vi "Swerve Drive Controller.vi"(8 "error in":errorcluster) -> ()   [LabVIEW 2016]
doc: "This VI executes continuously carrying out the current operation and responding to updates or new operations. It will often contain the timing or control code that is difficult to place directly in TeleOp. This VI generally opens all sensors and motors and isolates the rest of the robot code from knowing how the operations are carried out."
uses:
  Swerve Drive Setpoints.ctl
  Swerve Drive Operations.ctl
  <vilib>/Rock Robotics/WPI/ThirdParty/CanMotor/TalonSRX/WPI_CANTalonSRX_APIControlMode.ctl
  <vilib>/Rock Robotics/Network Tables/NT Read Boolean.vi
  Framework/Robot Global Data.vi
  Support Code/Team900-VIs/Team900SwerveDrive/SwerveDriveFuse.vi
  Swerve Drive Published Globals.vi
  <vilib>/Rock Robotics/Network Tables/SD Read Boolean.vi
  <vilib>/Rock Robotics/Network Tables/NT Read Numeric Array.vi
  Support Code/Team900-VIs/Team900SwerveDrive/SwerveGlobalData.vi
  Support Code/Team900-VIs/Team900SwerveDrive/Team900SwerveDrive.lvlib
  Support Code/Team900-VIs/navX Library v2/navX Library v2.lvlib
panel:
  in  "Reset Offsets":bool
  out "Loop Time":u32
  in  "Max Wheel Speed":dbl=20000.0
  in  "Distance PID gains":T1={"proportional gain (Kc)"=0.0125, "integral time (Ti, min)"=0.0, "derivative time (Td, min)"=0.00225} {"derivative time (Td, min)" format="%_5g"; "integral time (Ti, min)" format="%_5g"; "proportional gain (Kc)" format="%_5g"}
  in  "Face PID Gains":T1={"proportional gain (Kc)"=0.275, "integral time (Ti, min)"=0.0, "derivative time (Td, min)"=0.006} {"derivative time (Td, min)" format="%.3f"; "integral time (Ti, min)" format="%.3f"; "proportional gain (Kc)" format="%.3f"}
  out "Speed Chart":cluster{dbl, "Encoder Velocity":dbl}[](graph)
  out "Current\nCmd":string
  # "Tip: It may be helpful to observe inputs and sensor values.\nYou may also want to display tuning or debugging controls."
  # "To reset offsets, deploy the code, point the wheels facing toward the right of the robot, and the big gear facing to the back of the robot."
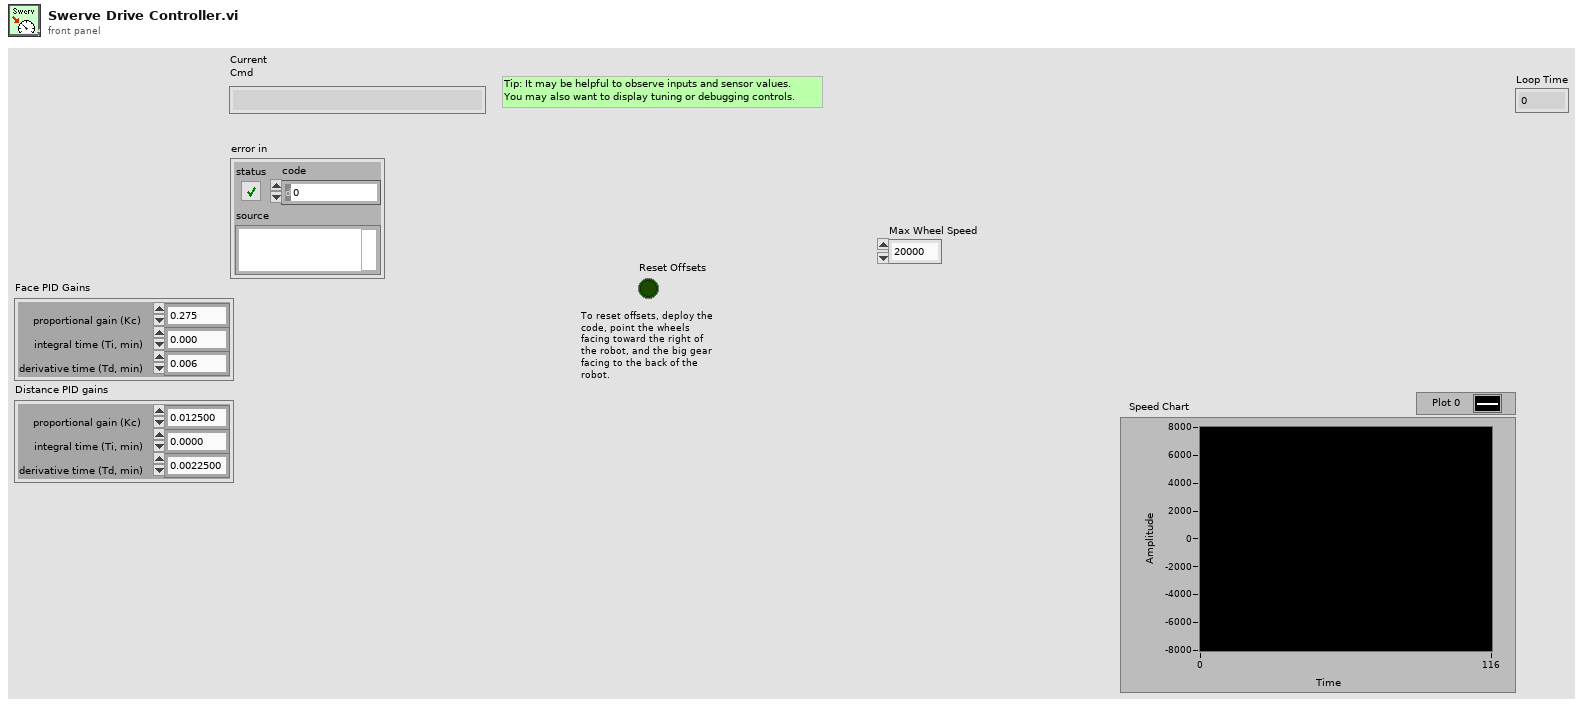
[diagram p1: front panel]
types:
  T1 = cluster{"proportional gain (Kc)":dbl, "integral time (Ti, min)":dbl, "derivative time (Td, min)":dbl}
  T2 = typedef "Swerve Drive Setpoints.ctl" = cluster{"Operation":T3, "Duration":dbl, "Strafe Joystick Axes":cluster{"X":dbl, "Y":dbl}, "Face Joystick Axes":cluster{"X":dbl, "Y":dbl}, "Trigger Axes":cluster{"Left":dbl, "Right":dbl}, "Coordinates":cluster{"X":dbl, "Y":dbl, "Angle":dbl}, "Speed Mode?":bool}
  T3 = typedef "Swerve Drive Operations.ctl" = enum16{"Reserve", "Read Current", "Immediate", "Go to Coordinate", "Drive Immediate (Turn Speed/Face and Stafe)"}
  T4 = typedef "Command Status Info.ctl" = cluster{"Name":string, "Status":T5, "notifier out":T6}
  T5 = typedef "Completion Status.ctl" = enum16{"Successful", "Aborted", "Incomplete"}
  T6 = typedef "Completion Notifier.ctl" = refnum<notifier>
  T7 = cluster{"Default Command":T2, "Command Timing":cluster{"Start Time (ms)":u32, "Iterations":i32}, "Command Arguments":cluster{"Command Info":T4, "Description":string, "Default Command":T2, "notifier out":refnum<notifier>, "Subsystem Name":string}}
  T8 = typedef "WPI_MotorControlDeviceRef.ctl" = cluster{"DeviceStatus":errorcluster, "Type":T9, "PWM":cluster{"PWM Channel":T10, "DeadBand":T11}, "CAN":cluster{"Device Number":u8, "SetOutput VI Ref":variant, "GetOutput VI Ref":variant, "Enable VI Ref":variant, "Disable VI Ref":variant, "Data":variant}, "Invert":bool}
  T9 = typedef "WPI_MotorControlType.ctl" = enum16{"PWM", "CAN"}
  T10 = typedef "FPGA_DIOPWMChannel.ctl" = enum8{"PWM 0", "PWM 1", "PWM 2", "PWM 3", "PWM 4", "PWM 5", "PWM 6", "PWM 7", "PWM 8", "PWM 9", "PWM MXP 0", "PWM MXP 1", "PWM MXP 2", "PWM MXP 3", "PWM MXP 4", "PWM MXP 5", "PWM MXP 6", "PWM MXP 7", "PWM MXP 8", "PWM MXP 9", "Invalid"}
  T11 = typedef "WPI_PWMDeadband.ctl" = cluster{"Name":string, "maxPositivePwm":i32, "minPositivePwm":i32, "centerPwm":i32, "maxNegativePwm":i32, "minNegativePwm":i32, "angularRange":u16}
  T12 = typedef "navX Library v2.lvlib/Z900_navX_DeviceTypeDef.ctl" = cluster{"Interface":cluster{"Protocol":T13, "Update Rate (4Hz-60Hz)":u8, "navX Open TypeDef":variant}, "Notify Packet":refnum<notifier>, "Loop VI Refnum":refnum<vi>, "Ready to Close Occurrence Refnum":refnum<k4>}
  T13 = typedef "navX Library v2.lvlib/Z900_navX_ProtocolTypeDef.ctl" = enum16{"SERIAL", "I2C", "SPI"}
  T14 = cluster{"Yaw":dbl, "Roll":dbl, "Pitch":dbl, "Heading":dbl, "Fused Heading":dbl}
  T15 = typedef "WPI_CANTalonSRX_GlobalStatus.ctl" = cluster{"Applied Throttle":dbl, "Module Enabled":bool, "CAN Error":errorcluster, "Closed Loop Error":dbl, "Forward Limit Switch Closed":bool, "Reverse Limit Switch Closed":bool, "Sensor Position":dbl, "Sensor Velocity":dbl, "Current":dbl, "Sticky Fault - Over Temp":bool, "Sticky Fault - Under Voltage":bool, "Sticky Fault - Forward Limit":bool, "Sticky Fault - Reverse Limit":bool, "Sticky Fault - Forward Soft Limit":bool, "Sticky Fault - Reverse Soft Limit":bool, "Brake is Enabled":bool, "Encoder Position":dbl, "Encoder Velocity":dbl, "Encoder Index Count":dbl, "Encoder A Pin State":bool, "Encoder B Pin State":bool, "Encoder Index Pin State":bool, "Analog In":dbl, "Analog In Velocity":dbl, "Temperature (C)":dbl, "Battery Voltage":dbl, "Control 5 Is Supported":bool, "Current Profile Slot Select":dbl, "Pos Div 8":bool, "Vel Div 4":bool, "Pulse Width Position":i32, "Pulse Width Velocity":i32, "Pulse Width Rise To Rise (us)":i32, "Pulse Width Rise To Fall (us)":i32, "Mot Prof Active Is Under Run":bool, "Mot Prof Active Has Under Run":bool, "Mot Prof Active Is Last":bool, "Mot Prof Active Velocity Only":bool, "Mot Prof Active Is Valid":bool, "Mot Prof Buffer Is Full":bool, "Mot Prof Active Profile Slot Select":i32, "Mot Prof NextID":i32, "Mot Prof Count":i32, "Mot Prof Active Velocity":dbl, "Mot Prof Active Position":dbl, "Mot Prof Output Enable":i32}
  T16 = cluster{"[0]":dbl, "[1]":dbl, "[2]":dbl, "[3]":dbl}
  T17 = cluster{"Numeric Array[0]":dbl, "Numeric Array[1]":dbl, "Numeric Array[2]":dbl}
  T18 = typedef "WPI_CANTalonSRX_APIControlMode.ctl" = enum8{"Percent VBus", "Speed", "Position", "Slave", "Unchanged / Invalid", "Voltage Compensation", "Current", "Motion Profile"}
  T19 = cluster{"Steering Motor Refs[0]":T8, "Steering Motor Refs[1]":T8, "Steering Motor Refs[2]":T8, "Steering Motor Refs[3]":T8}
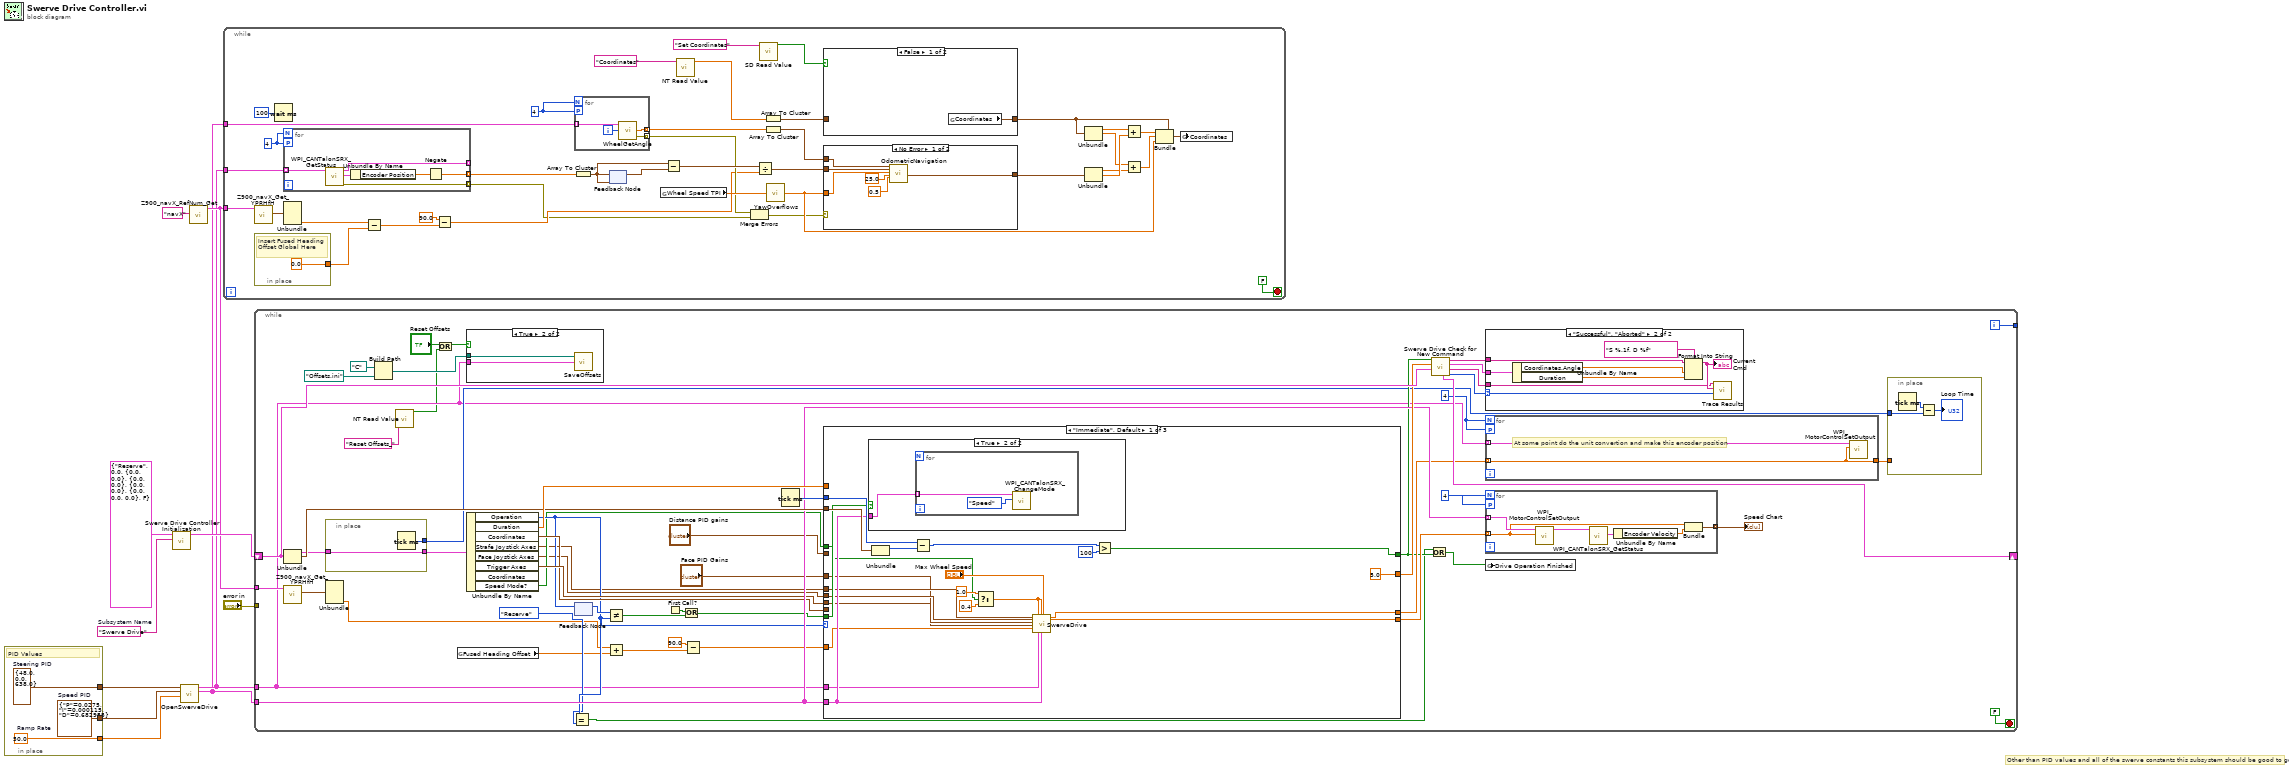
[diagram p0: block diagram]
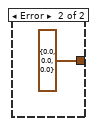
[diagram p2: hidden frame]
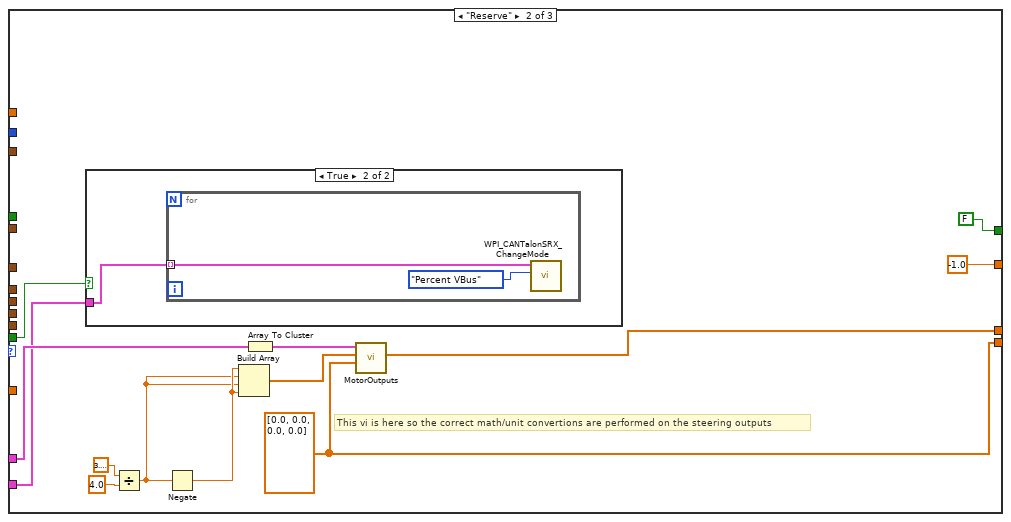
[diagram p7: hidden frame]
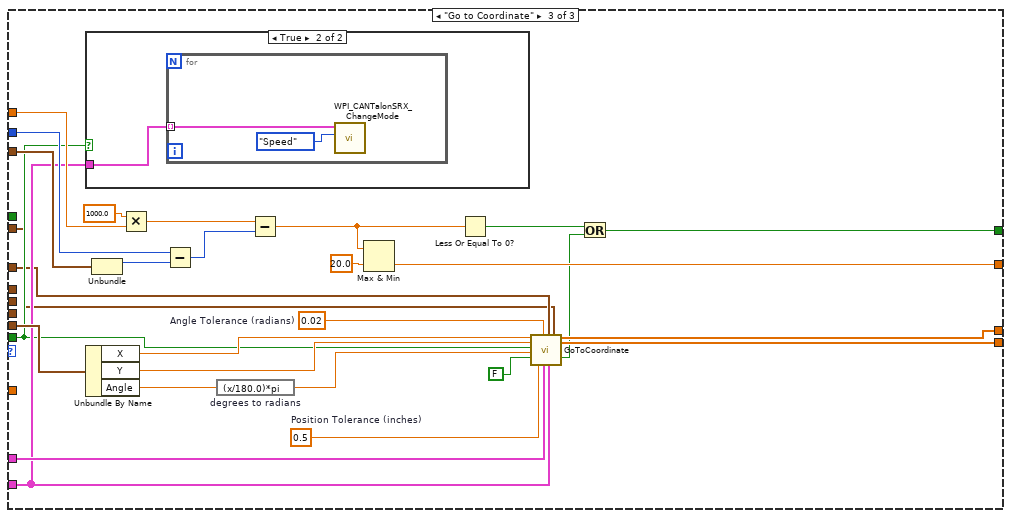
[diagram p9: hidden frame]
diagram:
  w1 = "Swerve Drive"  # Subsystem Name
  # "Other than PID values and all of the swerve constants this subsystem should be good to go"
  n1 = in-place {
    in-place-border: [w13] -> w9
    in-place-border: [w12] -> w8
    in-place-border: [w14] -> w4
    w14 = 50.0  # Ramp Rate
    w12 = cluster{"P":dbl, "I":dbl, "D":dbl} {"P"=0.0275, "I"=0.000115, "D"=0.682955}  # Speed PID
    w13 = cluster{"P":dbl, "I":dbl, "D":dbl} {"P"=48.0, "I"=0.0, "D"=638.0}  # Steering PID
    # "PID Values"
  }
  n2 = call "Swerve Drive Controller Initialization.vi"("Subsystem Name"=w1, "Default Command"=T2 {"Operation"=enum."Reserve", "Duration"=0.0, "Strafe Joystick Axes"={"X"=0.0, "Y"=0.0}, "Face Joystick Axes"={"X"=0.0, "Y"=0.0}, "Trigger Axes"={"Left"=0.0, "Right"=0.0}, "Coordinates"={"X"=0.0, "Y"=0.0, "Angle"=0.0}, "Speed Mode?"=FALSE}) -> ("Command Info"=w10:T7)  [unwired: 9 in]
  n3 = call "OpenSwerveDrive.vi"("Ramp Rate"=w4, "Speed PID"=w8, "Steering PID"=w9) -> ("Speed Motor Refs"=w2:T8[], "Steering Motor Refs"=w3:T8[])  [unwired: 4 in, 1 out]
  n4 = call "Z900_navX_RefNum_Get.vi"("refnum name"="navX") -> ("navX Device"=w6:T12)  [unwired: 9 in, 1 out]
  n5 = while {
    tunnel: w6 -> [w52]
    tunnel: w3 -> [w50]
    tunnel: w2 -> [w49]
    stop <- FALSE stop-if-true
    w23 = 4
    w24 = 4
    n6 = call "Z900_navX_Get_YPRHfH.vi"("navX Device"=w52) -> ("YRPHfH"=w48:T14)  [unwired: 7 in, 3 out]
    n7 = in-place {
      in-place-border: [0.0] -> w46
      # "Insert Fused Heading Offset Global Here"
    }
    n8 = Wait (ms)(milliseconds to wait=u32 100) -> ()  [unwired: 1 out]
    n9 = for {
      N: w24 -> [_]
      tunnel: [w68] -> _ mode=indexing
      tunnel: [w70] -> w34 mode=indexing
      workers-P: w24 -> [_]
      tunnel: w50 -> [w67] mode=indexing
      tunnel: [w66] -> w28 mode=indexing
      n10 = call <vilib>:"WPI_CANTalonSRX_GetStatus.vi"("CAN Talon SRX Ref"=w67) -> ("error out"=w70:errorcluster, "Talon SRX Status"=w69:T15, "CAN Talon SRX Ref"=w68:T8)  [unwired: 8 in]
      n11 = Unbundle By Name(w69) -> ("Encoder Position"=w65:dbl)
      n12 = Negate(x=w65) -> (-x=w66:dbl)
    }
    n13 = Unbundle(w48) -> ("Fused Heading"=w47:dbl)  [unwired: 4 out]
    n14 = Subtract(x=w47, y=w46) -> (x-y=w18:dbl)
    n15 = Subtract(x=90.0, y=w18) -> (x-y=w40:dbl)
    n16 = for {
      N: w23 -> [_]
      workers-P: w23 -> [_]
      tunnel: [w56] -> w27 mode=indexing
      tunnel: w49 -> [w55] mode=indexing
      tunnel: [w54] -> w25 mode=indexing
      i -> [w57]
      n17 = call "WheelGetAngle.vi"("Wheel"=w57, "CAN Talon SRX Ref"=w55) -> ("error out"=w56:errorcluster, "Sensor Position (rad)"=w54:dbl)  [unwired: 1 in, 1 out]
    }
    n18 = Array To Cluster(array=w28) -> (cluster=w29:T16)
    n19 = feedback #1(w29) -> (w30:T16)
    n20 = feedback-in #1(w29) -> ()
    n21 = global read "SwerveGlobalData.vi" "Wheel Speed TPI"() -> (w16:dbl)
    n22 = Subtract(x=w29, y=w30) -> (x-y=w31:T16)
    n23 = call-poly <vilib>:"NT Read Value.vi"("Name"="Coordinates") -> ("Numeric Array"=w22:dbl[])  [unwired: 9 in, 1 out]
    n24 = Merge Errors(w27, w34) -> (w33:errorcluster)
    n25 = Divide(x=w31, y=w16) -> (x/y=w32:T16)
    n26 = call-poly <vilib>:"SD Read Value.vi"("Name"="Set Coordinates") -> ("Boolean"=w19:bool)  [unwired: 8 in, 2 out]
    n27 = Array To Cluster(array=w22) -> (cluster=w21:T17)
    n28 = Array To Cluster(array=w25) -> (cluster=w26:T16)
    n29 = call "YawOverflows.vi"("Yaw (degrees)"=w40) -> ("Yaw (with overflows)"=w42:dbl)
    n30 = case shown="False" w19 {
      tunnel: [w71 w72] -> w45
      tunnel: w21 -> [_ w72]
      frame False {
        n31 = global read "SwerveGlobalData.vi" "Coordinates"() -> (w71:cluster{"X":dbl, "Y":dbl, "Heading":dbl})
      }
      frame True {
      }
    }
    n32 = case shown="No Error" w33 {
      tunnel: [w61 cluster{"sy":dbl, "sx":dbl, "rot.":dbl} {"sy"=0.0, "sx"=0.0, "rot."=0.0} ("movement")] -> w35
      tunnel: w32 -> [w63 _]
      tunnel: w26 -> [w62 _]
      tunnel: w42 -> [w58 _]
      frame No Error {
        n33 = call "OdometricNavigation.vi"("Wheel Angles (rad)"=w62, "Wheel Movements (in.)"=w63, "Robot angle (degrees)"=w58, "x and y error minimum (in.)"=25.0, "error minimum for rotation (rad)"=0.5 ("error minimum for rotation (in.)")) -> ("movement"=w61:cluster{"sy":dbl, "sx":dbl, "rot.":dbl})  [unwired: 14 in]
      }
      frame Error {
      }
    }
    n34 = Unbundle(w45) -> ("Numeric Array[0]"=w39:dbl, "Numeric Array[1]"=w37:dbl)  [unwired: 1 out]
    n35 = Unbundle(w35) -> ("sy"=w36:dbl, "sx"=w38:dbl)  [unwired: 1 out]
    n36 = Add(x=w39, y=w38) -> (x+y=w44:dbl)
    n37 = Add(x=w37, y=w36) -> (x+y=w43:dbl)
    n38 = Bundle(cluster=w45, "Numeric Array[0]"=w44, "Numeric Array[1]"=w43, "Numeric Array[2]"=w42) -> (w15:T17)
    n39 = global write "SwerveGlobalData.vi" "Coordinates"(w15) -> ()
  }
  n40 = while {
    shift-right: [w120] -> _
    shift-left: w10 -> [w121]
    tunnel: [w125] -> _
    tunnel: "error in" -> [_]
    tunnel: w3 -> [w83]
    tunnel: w2 -> [w111]
    tunnel: w6 -> [w94]
    i -> [w125]
    stop <- FALSE stop-if-true
    w112 = 4
    w113 = 4
    n41 = Unbundle(w121) -> ("Default Command"=w90:T2, "Command Timing"=w122:cluster{"Start Time (ms)":u32, "Iterations":i32})  [unwired: 1 out]
    n42 = call "Z900_navX_Get_YPRHfH.vi"("navX Device"=w94) -> ("YRPHfH"=w97:T14)  [unwired: 7 in, 3 out]
    n43 = in-place {
      in-place-border: w90 -> [w133]
      in-place-border: [w133] -> w89
      in-place-border: [w132] -> w87
      n44 = Tick Count (ms)() -> (millisecond timer value=w132:u32)
    }
    n45 = Unbundle(w97) -> ("Fused Heading"=w96:dbl)  [unwired: 4 out]
    n46 = Build Path(base path=path "C:/", name or relative path=path "Offsets.ini" ("default name")) -> (appended path=w84:path)
    n47 = call-poly <vilib>:"NT Read Value.vi"("Name"="Reset Offsets_") -> ("Boolean"=w74:bool)  [unwired: 9 in, 1 out]
    n48 = Or(x="Reset Offsets", y=w74) -> (x .or. y?=w75:bool)
    n49 = global read "Robot Global Data.vi" "Fused Heading Offset"() -> (w95:dbl)
    n50 = case shown="True" w75 {
      tunnel: w84 -> [_ w128]
      tunnel: w83 -> [_ w127]
      frame False {
      }
      frame True {
        n51 = call "SaveOffsets.vi"("CAN Talon SRX Ref"=w127, "configuration file path"=w128) -> ()  [unwired: 2 in, 1 out]
      }
    }
    n52 = Unbundle By Name(w89) -> ("Operation"=w100:T3, "Duration"=w124:dbl, "Coordinates"=w103:cluster{"X":dbl, "Y":dbl, "Angle":dbl}, "Strafe Joystick Axes"=w78:cluster{"X":dbl, "Y":dbl}, "Face Joystick Axes"=w77:cluster{"X":dbl, "Y":dbl}, "Trigger Axes"=w104:cluster{"Left":dbl, "Right":dbl}, "Speed Mode?"=w91:bool)  [unwired: 1 out]
    n53 = Equal?(x=w100, y=Swerve_Drive_Operations."Reserve") -> (x = y?=w98:bool)
    n54 = feedback-in #2(w100) -> ()
    n55 = feedback #2() -> (w108:T3)  [unwired: 1 in]
    n56 = Not Equal?(x=w108, y=w100) -> (x != y?=w107:bool)
    n57 = Add(x=w96, y=w95) -> (x+y=w80:dbl)
    n58 = First Call?() -> (First Call?: T/F=w106:bool)
    n59 = Or(x=w106, y=w107) -> (x .or. y?=w105:bool)
    n60 = Subtract(x=90.0, y=w80) -> (x-y=w79:dbl)
    n61 = Tick Count (ms)() -> (millisecond timer value=w123:u32)
    n62 = case shown="\"Immediate\", Default" w100 {
      tunnel: [5.0 -1.0 w207] -> w119
      tunnel: [w166 FALSE ("ignore previous (F)") w210] -> w102
      tunnel: w122 -> [w168 _ w218]
      tunnel: w124 -> [_ _ w215]
      tunnel: w123 -> [w167 _ w216]
      tunnel: w83 -> [w155 w179 w199]
      tunnel: w111 -> [w162 w176 w194]
      tunnel: [w165 w180 w197] -> w110
      tunnel: [w164 w175 w198] -> w109
      tunnel: w105 -> [w163 w177 w193]
      tunnel: w78 -> [w161 _ _]
      tunnel: w77 -> [w160 _ _]
      tunnel: w104 -> [w159 _ _]
      tunnel: w103 -> [_ _ w206]
      tunnel: w79 -> [w158 _ _]
      tunnel: "Face PID Gains" -> [w157 _ w192]
      tunnel: "Distance PID gains" -> [_ _ w191]
      tunnel: w91 -> [w151 _ _]
      frame "Immediate", Default {
        n63 = case shown="True" w163 {
          tunnel: w162 -> [_ w172]
          frame False {
          }
          frame True {
            n64 = for {
              tunnel: w172 -> [w174] mode=indexing
              n65 = call <vilib>:"WPI_CANTalonSRX_ChangeMode.vi"("Control Mode"=WPI_CANTalonSRX_APIControlMode."Speed", "CAN Talon SRX Ref"=w174) -> ()  [unwired: 8 in, 2 out]
            }
          }
        }
        n66 = Unbundle(w168) -> ("Start Time (ms)"=w171:u32)  [unwired: 1 out]
        n67 = Subtract(x=w167, y=w171) -> (x-y=w170:u32)
        n68 = Select(t=1.0 ("Rotation Multiplier"), s=w151, f=0.4) -> (s? t:f=w153:dbl)
        n69 = call-poly "SwerveDrive.vi"("Strafe Joystick Axes"=w161, "Face Joystick Axes"=w160, "Trigger Axes"=w159, "Face PID Gains"=w157, "Angle (degrees; 0 = right)"=w158, "Strafe Multiplier"=w153, "Steering Motor Refs"=w155, "Rotation Multiplier"=w153, "Speed Motor Refs"=w162, "Max Wheel Speed"="Max Wheel Speed") -> ("Steering Motor Setpoints"=w165:dbl[], "Speed Motor Setpoints"=w164:dbl[])  [unwired: 6 in, 2 out]
        n70 = Greater?(x=w170, y=u8 100 ("Left Motor")) -> (0:w166:bool)
      }
      frame "Reserve" {
        w175 = dbl[] [0.0, 0.0, 0.0, 0.0] ("appended array")
        # "This vi is here so the correct math/unit convertions are performed on the steering outputs"
        n71 = case shown="True" w177 {
          tunnel: w176 -> [_ w188]
          frame False {
          }
          frame True {
            n72 = for {
              tunnel: w188 -> [w190] mode=indexing
              n73 = call <vilib>:"WPI_CANTalonSRX_ChangeMode.vi"("Control Mode"=WPI_CANTalonSRX_APIControlMode."Percent VBus", "CAN Talon SRX Ref"=w190) -> ()  [unwired: 8 in, 2 out]
            }
          }
        }
        n74 = Divide(x=3.141592653589793, y=4.0) -> (x/y=w184:dbl)
        n75 = Negate(x=w184) -> (-x=w185:dbl)
        n76 = Build Array(w185, w184, w184, w185) -> (w181:dbl[])
        n77 = Array To Cluster(array=w179) -> (cluster=w178:T19)
        n78 = call "MotorOutputs.vi"("Motor Speeds"=w175, "Target Angles"=w181, "Steering Refnums In"=w178) -> ("Steering Motor Setpoints"=w180:dbl[])  [unwired: 5 in, 3 out]
      }
      frame "Go to Coordinate" {
        w200 = 0.02  # Angle Tolerance (radians)
        w201 = 0.5  # Position Tolerance (inches)
        n79 = case shown="True" w193 {
          tunnel: w194 -> [_ w219]
          frame False {
          }
          frame True {
            n80 = for {
              tunnel: w219 -> [w221] mode=indexing
              n81 = call <vilib>:"WPI_CANTalonSRX_ChangeMode.vi"("Control Mode"=WPI_CANTalonSRX_APIControlMode."Speed", "CAN Talon SRX Ref"=w221) -> ()  [unwired: 8 in, 2 out]
            }
          }
        }
        n82 = Unbundle By Name(w206) -> ("X"=w205:dbl, "Y"=w204:dbl, "Angle"=w195:dbl)
        n83 = Unbundle(w218) -> ("Start Time (ms)"=w217:u32)  [unwired: 1 out]
        n84 = Multiply(x=1000.0, y=w215) -> (x*y=w213:dbl)
        n85 = Subtract(x=w216, y=w217) -> (x-y=w212:u32)
        n86 = expression code="(x/180.0)*pi" "degrees to radians"(w195) -> (w203:dbl)
        n87 = Subtract(x=w213, y=w212) -> (x-y=w209:dbl)
        n88 = Max & Min(x=w209, y=20.0) -> (min(x,y)=w207:dbl)  [unwired: 1 out]
        n89 = Less Or Equal To 0?(x=w209) -> (x <= 0?=w211:bool)
        n90 = call "GoToCoordinate.vi"("Target X"=w205, "Target Y"=w204, "Reset (for robot centric)"=w193, "Target Angle (rad)"=w203, "Field Centric?"=FALSE, "Position Tolerance"=w201, "Angle Tolerance"=w200, "Steering Motor Refs"=w199, "Face PID Gains"=w192, "Speed Motor Refs"=w194, "Distance PID gains"=w191) -> ("Steering Motor Setpoints"=w197:dbl[], "Speed Motor Setpoints"=w198:dbl[], "Finished"=w196:bool)  [unwired: 5 in, 1 out]
        n91 = Or(x=w211, y=w196) -> (x .or. y?=w210:bool)
      }
    }
    n92 = Or(x=w98, y=w102) -> (x .or. y?=w101:bool)
    n93 = call "Swerve Drive Check for New Command.vi"("Current Command"=w121, "Wait time (ms)"=w119, "Finished?"=w102) -> ("Completion"=w115:T5, "Subsystem Name"=w116:string, "Current Command"=w117:T2, "Initial Trace String"=w118:string, "NextCommand"=w120:T7)  [unwired: 4 in]
    n94 = case shown="\"Successful\", \"Aborted\"" w115 {
      selector: w115 -> [_ w149]
      tunnel: w118 -> [_ w145]
      tunnel: w117 -> [_ w146]
      tunnel: w116 -> [_ w142]
      frame "Incomplete", Default {
        # "Continuing current command"
      }
      frame "Successful", "Aborted" {
        # "Report and setup for next command"
        n95 = Unbundle By Name(w146) -> ("Coordinates.Angle"=w148:dbl, "Duration"=w143:dbl)
        n96 = Format Into String(format string="S %.1f, D %f", initial string=w145, w148, w143) -> (resulting string=w144:string)  [unwired: 1 in, 1 out]
        "Current\nCmd" <- w144
        n97 = call <vilib>:"Trace Results.vi"("Status of previous command"=w149, "Description"=w144, "Subsystem"=w142) -> ()  [unwired: 9 in]
      }
    }
    n98 = for {
      N: w112 -> [_]
      workers-P: w112 -> [_]
      tunnel: w83 -> [w141] mode=indexing
      tunnel: w110 -> [w140] mode=indexing
      tunnel: [w140] -> w88
      # "At some point do the unit convertion and make this encoder position"
      n99 = call <vilib>:"WPI_MotorControlSetOutput.vi"("Output"=w140, "MotorControlDevRef"=w141) -> ()  [unwired: 7 in, 3 out]
    }
    n100 = for {
      N: w113 -> [_]
      workers-P: w113 -> [_]
      tunnel: w111 -> [w139] mode=indexing
      tunnel: w109 -> [w134] mode=indexing
      tunnel: [w135] -> w114 mode=indexing
      n101 = call <vilib>:"WPI_MotorControlSetOutput.vi"("Output"=w134, "MotorControlDevRef"=w139) -> ("MotorControlDevRef"=w137:T8)  [unwired: 7 in, 2 out]
      n102 = call <vilib>:"WPI_CANTalonSRX_GetStatus.vi"("CAN Talon SRX Ref"=w137) -> ("Talon SRX Status"=w138:T15)  [unwired: 8 in, 2 out]
      n103 = Unbundle By Name(w138) -> ("Encoder Velocity"=w136:dbl)
      n104 = Bundle(w134, "Encoder Velocity"=w136) -> (w135:cluster{dbl, "Encoder Velocity":dbl})  [unwired: 1 in]
    }
    "Speed Chart" <- w114
    n105 = global write "Swerve Drive Published Globals.vi" "Drive Operation Finished"(w101) -> ()
    n106 = in-place {
      in-place-border: w88 -> [_]
      in-place-border: w87 -> [w130]
      n107 = Tick Count (ms)() -> (millisecond timer value=w131:u32)
      n108 = Subtract(x=w131, y=w130) -> (x-y=→"Loop Time":u32)
    }
  }
